vi "Get_Parent_Panel.vi"(8 "error in (no error)":errorcluster, 11 "Child_Panel in":refnum<class "Panel2.lvclass">) -> (0 "error out":errorcluster, 1 "Status":bool, 2 "Parent_Panel":refnum<class "Panel_Interface.lvclass">, 3 "Child_Panel out":refnum<class "Panel2.lvclass">)   [LabVIEW 2021, in "Panel2.lvclass"]
uses:
  Panel2.lvclass
  C:/Program Files (x86)/Hyper State Machine Framework/SSW_Panel_Adaptive.lvlibp/Panel_Interface/Panel_Interface.lvclass
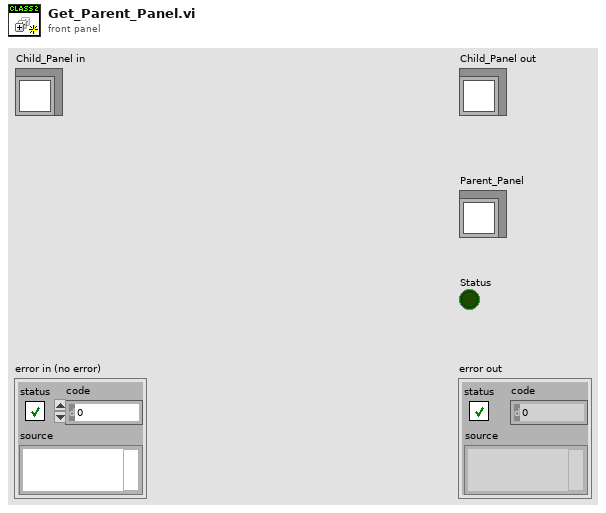
[diagram p1: front panel]
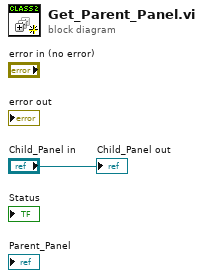
[diagram p0: block diagram]
diagram:
  "Child_Panel out" <- "Child_Panel in"
